vi "Write CSV File (UTF-16).vi"   [LabVIEW 2013, in "SET_Robust CSV (UTF-16).lvlib"]
uses:
  SET_Robust CSV (UTF-16).lvlib
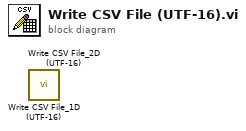
[diagram p0: block diagram]
diagram:
  n1 = call "Write CSV File_1D (UTF-16).vi"() -> ()  [unwired: 10 in, 2 out]
  n2 = call "Write CSV File_2D (UTF-16).vi"() -> ()  [unwired: 10 in, 2 out]
